vi "CDMA_RxTimeslotSyn.vi"(7 "corr_length":dbl, 8 "error in (no error)":errorcluster caption="错误输入（无错误）", 9 "sampleRate":dbl, 10 "rx_data":cdb[](array[numeric]), 11 "Path In":path) -> (0 "error out":errorcluster caption="错误输出", 1 "timeslot_star":dbl, 2 "searchFlag":dbl, 3 "Path Out":path, 4 "PscCorr":dbl[](array[numeric]))   [LabVIEW 2015]
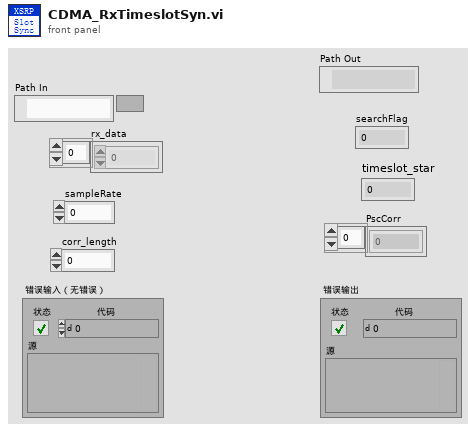
[diagram p1: front panel]
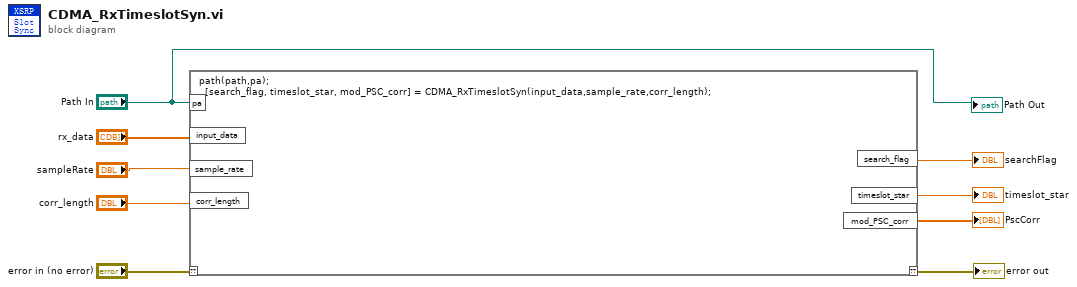
[diagram p0: block diagram]
diagram:
  n1 = script code="path(path,pa);\n  [search_flag, timeslot_star, mod_PSC_corr] = CDMA_RxTimeslotSyn(input_data,sample_rate,corr_length);"("??"="error in (no error)", "pa"="Path In", "input_data"="rx_data", "sample_rate"="sampleRate", "corr_length"="corr_length") -> ("??"=→"error out":errorcluster, "search_flag"=→"searchFlag":dbl, "timeslot_star"=→"timeslot_star":dbl, "mod_PSC_corr"=→"PscCorr":dbl[])
  "Path Out" <- "Path In"
